vi "arrow keys.vi"() -> ()   [LabVIEW 2023]
panel:
  in  "Filter":string
  in  "Listbox":i32(listbox)
  # "Down arrow selects first item\nOn last item down arrow goes ot first item\nOn first item up arrow goes to filter"
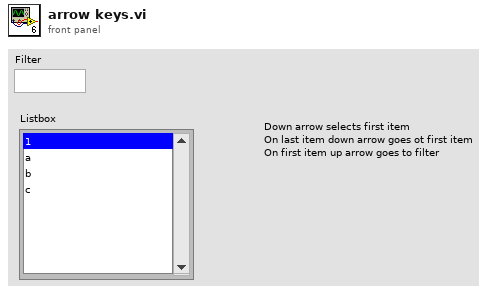
[diagram p1: front panel]
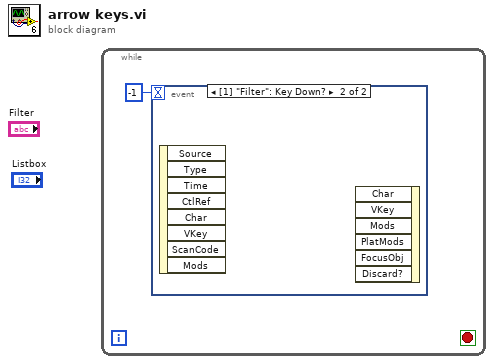
[diagram p0: block diagram]
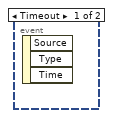
[diagram p2: hidden frame]
diagram:
  n1 = while {
    stop <- _ stop-if-true
    n2 = event shown="[1] \"Filter\": Key Down?" {
      selector: _ -> [_ _]
      dyn-events: _ -> [_ _]
      timeout: -1 -> [_ _]
      event Timeout {
        n3 = event-data() -> ()  [unwired: 1 in, 3 out]
      }
      event "Filter": Key Down? {
        n4 = event-data() -> ()  [unwired: 1 in, 8 out]
        n5 = event-data() -> ()  [unwired: 7 in, 1 out]
      }
    }
  }
